vi "gfitsio-get-current-hdu-info.vi"(8 "error in (no error)":errorcluster, 11 "gfits refnum":T2) -> (0 "error out":errorcluster, 1 "hdu number":i32, 2 "hdu name":string, 3 "dup gfits refnum":T2, 4 "hdu type":T1 items=["ANY_HDU"=-1, "IMAGE_HDU"=0, "ASCII_TBL"=1, "BINARY_TBL"=2])   [LabVIEW 2019, in "gfitsio.lvlib"]
doc: "Return the number of the current HDU (CHDU) in the FITS file (where the primary array = 1), the name of the CHDU (if it is stored in the EXTNAME keyword), and the type of the CHDU in the FITS file."
uses:
  gfitsio.lvlib
  gfitsio-refnum.ctl
  cfitsio-hdutypes.ctl
  <vilib>/Utility/error.llb/DialogType.ctl
  gfitsio.dll
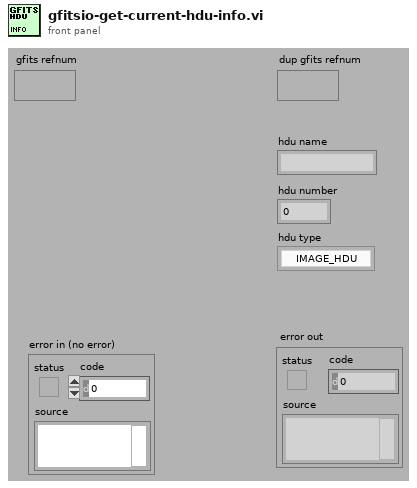
[diagram p1: front panel]
types:
  T1 = typedef "gfitsio.lvlib/cfitsio-hdutypes.ctl" = i32
  T2 = typedef "gfitsio.lvlib/gfitsio-refnum.ctl" = refnum<k1>
  T3 = typedef "DialogType.ctl" = u16
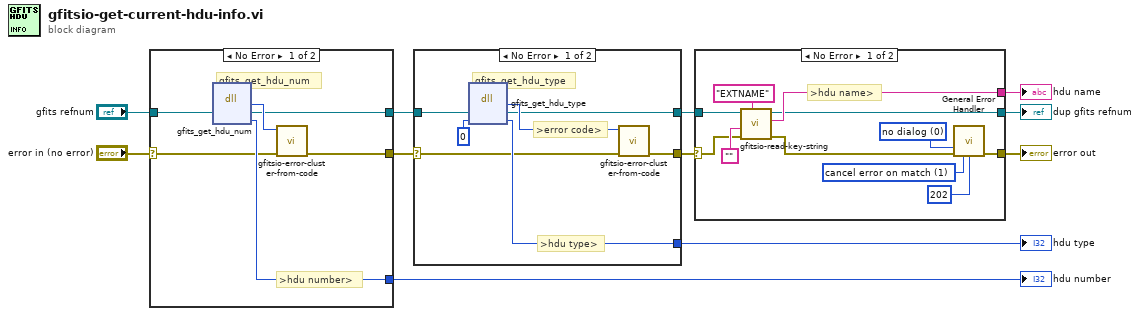
[diagram p0: block diagram]
diagram:
  n1 = case shown="No Error" "error in (no error)" {
    selector: "error in (no error)" -> [w15 w19]
    tunnel: [w14 w19] -> w5
    tunnel: "gfits refnum" -> [w12 w18]
    tunnel: [w13 w18] -> w6
    tunnel: [w17 _] -> w9
    frame No Error {
      # "gfits_get_hdu_num"
      # ">hdu number>"
      n2 = dll-call lib="C:/Users/ggatling/local/GFITSIO/gfitsio/gfitsio.dll" fn="gfits_get_hdu_num"("gfits refnum"=w12) -> (w16:i32, "gfits refnum"=w13:T2, "hdunum"=w17:i32)  [unwired: 3 in, 3 out]
      n3 = call "gfitsio-error-cluster-from-code.vi"("error in (no error)"=w15, "error code"=w16) -> ("error out"=w14:errorcluster)  [unwired: 9 out]
    }
    frame Error {
    }
  }
  "hdu number" <- w9
  n4 = case shown="No Error" w5 {
    selector: w5 -> [w24 w28]
    tunnel: [w23 w28] -> w1
    tunnel: w6 -> [w21 w27]
    tunnel: [w22 w27] -> w4
    tunnel: [w26 _] -> w7
    frame No Error {
      # ">hdu type>"
      # ">error code>"
      # "gfits_get_hdu_type"
      n5 = dll-call lib="C:/Users/ggatling/local/GFITSIO/gfitsio/gfitsio.dll" fn="gfits_get_hdu_type"("gfits refnum"=w21, "hdunum"=0) -> (w25:i32, "gfits refnum"=w22:T2, "hdunum"=w26:i32)  [unwired: 3 in, 2 out]
      n6 = call "gfitsio-error-cluster-from-code.vi"("error in (no error)"=w24, "error code"=w25) -> ("error out"=w23:errorcluster)  [unwired: 9 out]
    }
    frame Error {
    }
  }
  "hdu type" <- w7
  n7 = case shown="No Error" w1 {
    selector: w1 -> [w29 w40]
    tunnel: [w38 _] -> w8
    tunnel: w4 -> [w37 w41]
    tunnel: [w31 w40] -> w3
    tunnel: [w30 w41] -> w2
    frame No Error {
      w32 = T3 0 items=["no dialog", "OK message", "continue or stop message", "OK message + warnings", "continue/stop + warnings"] ("type of dialog (OK msg:1)")
      w33 = 1 items=["no exception", "cancel error on match", "set error on match"] ("[exception action] (none:0)")
      # ">hdu name>"
      n8 = call "gfitsio-read-key-string.vi"("keyname"="EXTNAME", "error in (no error)"=w29, "default value"="", "gfits refnum"=w37) -> ("error out"=w39:errorcluster, "value"=w38:string, "dup gfits refnum"=w30:T2)  [unwired: 1 in, 4 out]
      n9 = call <vilib>:"General Error Handler.vi"("type of dialog (OK msg:1)"=w32, "error in (no error)"=w39, "[exception action] (none:0)"=w33, "[exception code]"=202) -> ("error out"=w31:errorcluster)  [unwired: 1 in, 10 out]
    }
    frame Error {
    }
  }
  "error out" <- w3
  "dup gfits refnum" <- w2
  "hdu name" <- w8
